vi "UDP Send (core).vi"(7 "timeout ms (100)":i32=100, 8 "error in (no error)":errorcluster, 9 "Data":string, 10 "IP":string, 11 "connection ID in":refnum<k16>) -> (0 "error out":errorcluster, 3 "connection ID out":refnum<k16>)   [LabVIEW 2016, in "SMD-7615.lvlib" / "eSCL.lvlib"]
uses:
  eSCL.lvlib
panel:
  out "send string":string
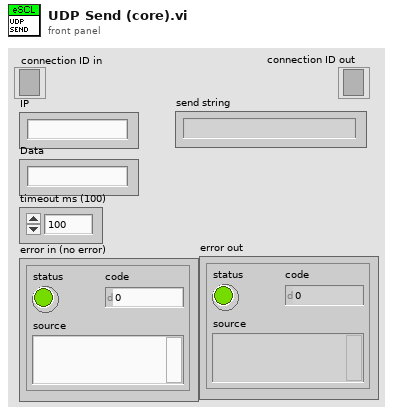
[diagram p1: front panel]
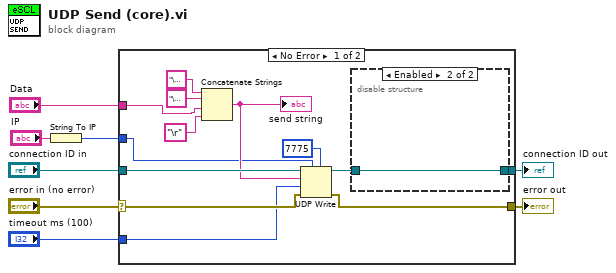
[diagram p0: block diagram]
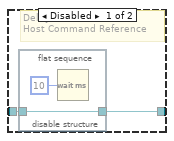
[diagram p2: hidden frame]
diagram:
  n1 = String To IP(1:"IP") -> (0:w2:u32)
  n2 = case shown="No Error" "error in (no error)" {
    selector: "error in (no error)" -> [w18 w27]
    tunnel: "connection ID in" -> [w20 w28]
    tunnel: [w9 w28] -> w6
    tunnel: [w19 w27] -> w5
    tunnel: "Data" -> [w14 _]
    tunnel: w2 -> [w12 _]
    tunnel: "timeout ms (100)" -> [w11 _]
    frame No Error {
      n3 = Concatenate Strings("\u0000" ("string"), "\u0007" ("string"), w14, "\r" ("string")) -> (w13:string)
      "send string" <- w13
      n4 = UDP Write(address=w12, port or service name=u16 7775 ("port"), connection ID=w20, data in=w13, 8:w18, 9:w11) -> (error out=w19:errorcluster, 3:w10:refnum<k16>)
      n5 = disable-structure shown="Enabled" {
        disable-tunnel: w10 -> [w23 w26]
        disable-tunnel: [w22 w26] -> w9
        frame Disabled {
          # "Delay is advised in \nHost Command Reference"
          n6 = flat-sequence {
            tunnel: [w24] -> w22
            tunnel: w23 -> [w24]
            frame #0 {
              n7 = Wait (ms)(milliseconds to wait=u32 10) -> ()  [unwired: 1 out]
            }
          }
        }
        frame Enabled {
        }
      }
    }
    frame Error {
    }
  }
  "connection ID out" <- w6
  "error out" <- w5
